vi "Pressure.vi"(8 "error in (no error)":errorcluster, 10 "Pressure":dbl, 11 "VISA resource name":refnum<visa-resource-name>) -> (0 "error out":errorcluster, 3 "VISA resource name out":refnum<visa-resource-name>)   [LabVIEW 2021, in "Dispenser.lvclass"]
uses:
  Dispenser.lvclass
  Drivers/EFD Ultimus V/EFD Ultimus V.lvlib
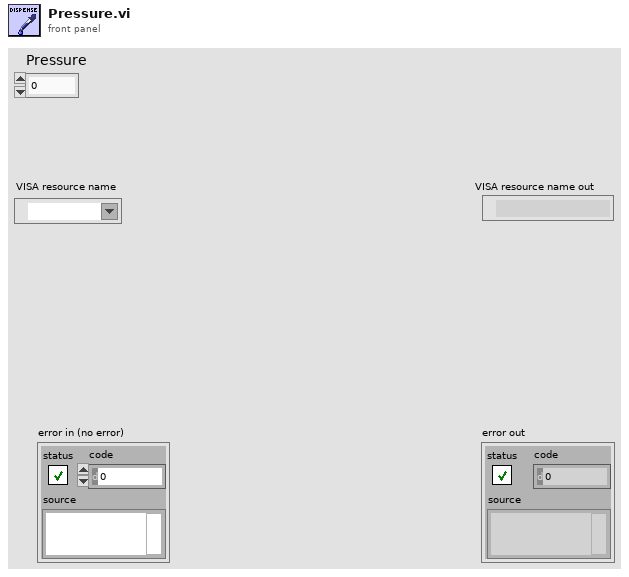
[diagram p1: front panel]
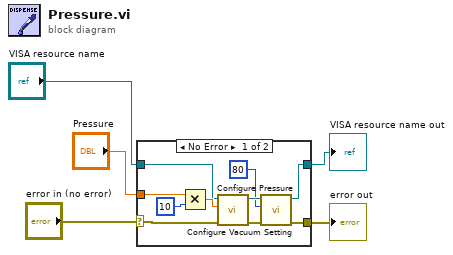
[diagram p0: block diagram]
diagram:
  n1 = case shown="No Error" "error in (no error)" {
    selector: "error in (no error)" -> [w11 w17]
    tunnel: [w8 w17] -> w4
    tunnel: "Pressure" -> [w14 _]
    tunnel: "VISA resource name" -> [w12 w16]
    tunnel: [w9 w16] -> w2
    frame No Error {
      n2 = Multiply(x=w14, y=i16 10) -> (x*y=w13:dbl)
      n3 = call "Configure Pressure.vi"("error in (no error)"=w11, "Pressure Setting (0000)"=w13, "VISA resource name"=w12) -> ("error out"=w7:errorcluster, "VISA resource name out"=w10:refnum<visa-resource-name>)  [unwired: 7 in]
      n4 = call "Configure Vacuum Setting.vi"("error in (no error)"=w7, "Vacuum Setting (0000)"=i64 80, "VISA resource name"=w10) -> ("error out"=w8:errorcluster, "VISA resource name out"=w9:refnum<visa-resource-name>)  [unwired: 7 in]
    }
    frame Error {
    }
  }
  "error out" <- w4
  "VISA resource name out" <- w2
